vi "Elapsed_time.vi"(6 "Elapsed time (s)":dbl, 7 "Inner N":i32, 8 "Inner i":i32, 9 "Outer i":i32, 10 "Front_panel_refs":T1, 11 "Outer N":i32) -> (2 "Front_panel_refs out":T1)   [LabVIEW 2016]
uses:
  Front_panel_refs.ctl
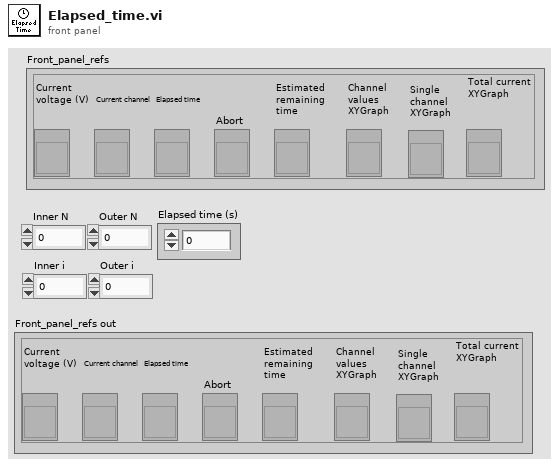
[diagram p1: front panel]
types:
  T1 = typedef "Front_panel_refs.ctl" = cluster{"Current voltage (V)":refnum<vi>, "Elapsed time":refnum<vi>, "Current channel":refnum<vi>, "Abort":refnum<vi>, "Estimated remaining time":refnum<vi>, "Channel values XYGraph":refnum<vi>, "Single channel XYGraph":refnum<vi>, "Total current XYGraph":refnum<vi>}
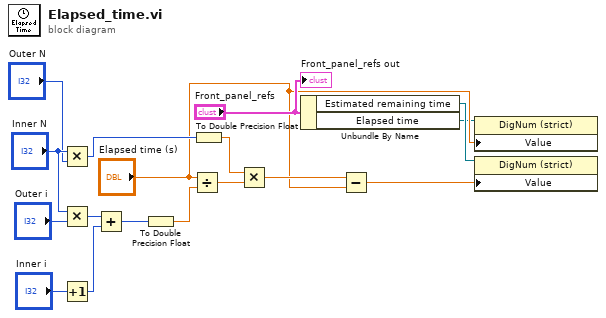
[diagram p0: block diagram]
diagram:
  n1 = Multiply(x="Inner N", y="Outer N") -> (x*y=w12:i32)
  n2 = Multiply(x="Inner N", y="Outer i") -> (x*y=w15:i32)
  n3 = Increment(x="Inner i") -> (x+1=w14:i32)
  n4 = Add(x=w15, y=w14) -> (x+y=w10:i32)
  n5 = To Double Precision Float(number=w10) -> (double precision float=w9:dbl)
  n6 = Divide(x="Elapsed time (s)", y=w9) -> (x/y=w17:dbl)
  n7 = To Double Precision Float(number=w12) -> (double precision float=w11:dbl)
  n8 = Multiply(x=w11, y=w17) -> (x*y=w16:dbl)
  n9 = Unbundle By Name("Front_panel_refs") -> ("Estimated remaining time"=w8:refnum<vi>, "Elapsed time"=w1:refnum<vi>)
  n10 = Subtract(x=w16, y="Elapsed time (s)") -> (x-y=w13:dbl)
  n11 = property class="DigNum (strict)"(reference=w1, "Value"="Elapsed time (s)") -> ()  [unwired: 1 in, 2 out]
  n12 = property class="DigNum (strict)"(reference=w8, "Value"=w13) -> ()  [unwired: 1 in, 2 out]
  "Front_panel_refs out" <- "Front_panel_refs"
